vi "Cleanup (User).vi"(8 "error in":errorcluster, 11 "Node in":refnum<class "BLS Power Supply Template.lvclass">) -> (0 "error out":errorcluster caption="error in", 3 "Node out":refnum<class "BLS Power Supply Template.lvclass">)   [LabVIEW 2023, in "BLS Power Supply Template.lvlib" / "BLS Power Supply Template.lvclass"]
uses:
  BLS Power Supply Template.lvclass
  BLS Power Supply Template.lvclass/BLS Power Supply Template.ctl
  bls-capabilities/src/Capabilities/High Level Capabilities/Power Supply/Power Supply.lvclass
  bls-capabilities/src/Capabilities/High Level Capabilities/Power Supply/Output Enable Write Single.vi
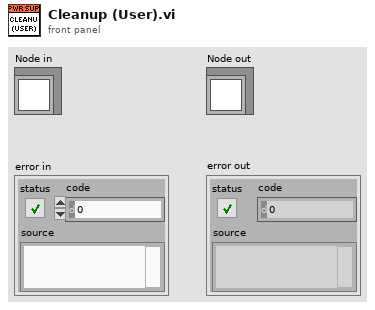
[diagram p1: front panel]
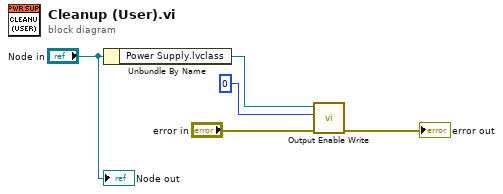
[diagram p0: block diagram]
diagram:
  n1 = Unbundle By Name("Node in") -> ("Power Supply.lvclass"=w2:refnum<class "Power Supply.lvclass">)
  n2 = call-poly "Output Enable Write.vi"("error in"="error in", "Output Enable STS"=0, "Power Supply In"=w2) -> ("error out"=→"error out":errorcluster)  [unwired: 7 in, 1 out]
  "Node out" <- "Node in"
